vi "PicoScope3000aSettings.vi"(0 "handle in":i16, 1 "Channel A Settings":T1={"Enabled"=FALSE, "Coupling"=1, "Range"=6, "Analogue Offset"=0.0, "Bandwidth Limit"=0} {"Bandwidth Limit" items=["Full", "20MHz"]; "Range" items=["10 mV", "20 mV", "50 mV", "100 mV", "200 mV", "500 mV", "1 V", "2 V", "5 V", "10 V", "20 V", "50 V ", "100 V"]; "Coupling" items=["AC", "DC"]}, 2 "Channel B Settings":T1={"Enabled"=FALSE, "Coupling"=1, "Range"=6, "Analogue Offset"=0.0, "Bandwidth Limit"=0} {"Bandwidth Limit" items=["Full", "20MHz"]; "Range" items=["10 mV", "20 mV", "50 mV", "100 mV", "200 mV", "500 mV", "1 V", "2 V", "5 V", "10 V", "20 V", "50 V ", "100 V"]; "Coupling" items=["AC", "DC"]}, 3 "Port 0 Settings":T4={"Enabled"=FALSE, "Logic Level"=9830} {"Logic Level" items=["1.5V TTL"=9830, "2.5V CMOS"=16383]}, 5 "Trigger Settings":T3={"Trigger Enabled"=FALSE, "Trigger Source"=enum."Channel A", "Trigger Threshold (volts)"=0.0, "Trigger Direction"=2, "Trigger Delay (samples)"=0, "Auto Trigger Time (ms)"=1000} {"Trigger Direction" items=["Above", "Below", "Rising", "Falling", "Rising or Falling"]}, 7 "Max_adc":i16=32767, 9 "Device Info":T2, 11 "error in":errorcluster, 12 "Channel C Settings":T1={"Enabled"=FALSE, "Coupling"=1, "Range"=6, "Analogue Offset"=0.0, "Bandwidth Limit"=0} {"Bandwidth Limit" items=["Full", "20MHz"]; "Range" items=["10 mV", "20 mV", "50 mV", "100 mV", "200 mV", "500 mV", "1 V", "2 V", "5 V", "10 V", "20 V", "50 V ", "100 V"]; "Coupling" items=["AC", "DC"]}, 13 "Channel D Settings":T1={"Enabled"=FALSE, "Coupling"=1, "Range"=6, "Analogue Offset"=0.0, "Bandwidth Limit"=0} {"Bandwidth Limit" items=["Full", "20MHz"]; "Range" items=["10 mV", "20 mV", "50 mV", "100 mV", "200 mV", "500 mV", "1 V", "2 V", "5 V", "10 V", "20 V", "50 V ", "100 V"]; "Coupling" items=["AC", "DC"]}, 14 "Port 1 Settings":T4={"Enabled"=FALSE, "Logic Level"=9830} {"Logic Level" items=["1.5V TTL"=9830, "2.5V CMOS"=16383]}) -> (4 "handle out":i16, 8 "Enabled Array":i16[](array[numeric]), 15 "error out":errorcluster)   [LabVIEW 2010]
doc: "This VI is used to set up the oscilloscope channels and call the SetSimpleTrigger function."
uses:
  ps3000a.dll
  PicoScope3000aAnalogChannelSettings.ctl
  PicoScope3000aDigitalChannelSettings.ctl
panel:
  # "Connect to PicoScope3000aOpen.vi"
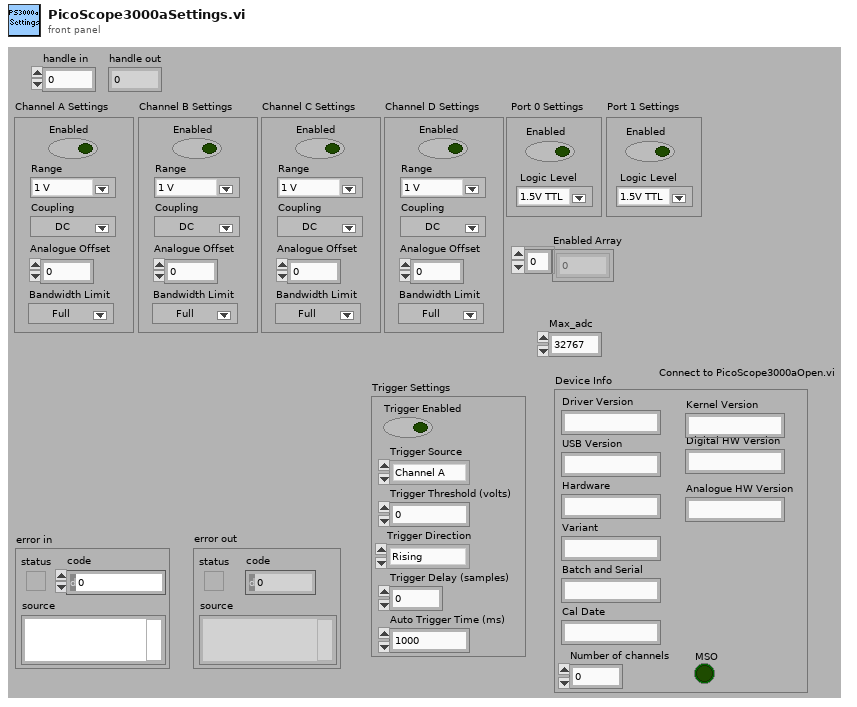
[diagram p1: front panel]
types:
  T1 = typedef "PicoScope3000aAnalogChannelSettings.ctl" = cluster{"Enabled":bool, "Coupling":u32, "Range":u32, "Analogue Offset":sgl, "Bandwidth Limit":u32}
  T2 = cluster{"Driver Version":string, "USB Version":string, "Hardware":string, "Variant":string, "Batch and Serial":string, "Cal Date":string, "Kernel Version":string, "Digital HW Version":string, "Analogue HW Version":string, "MSO":bool, "Number of channels":i16}
  T3 = cluster{"Trigger Enabled":bool, "Trigger Source":enum32{"Channel A", "Channel B", "Channel C", "Channel D", "Ext."}, "Trigger Threshold (volts)":dbl, "Trigger Direction":u32, "Trigger Delay (samples)":u32, "Auto Trigger Time (ms)":i16}
  T4 = typedef "PicoScope3000aDigitalChannelSettings.ctl" = cluster{"Enabled":bool, "Logic Level":i16}
  T5 = cluster{"status":bool, "code":u32, "source":string}
  T6 = enum32{"Channel A", "Channel B", "Channel C", "Channel D", "Ext."}
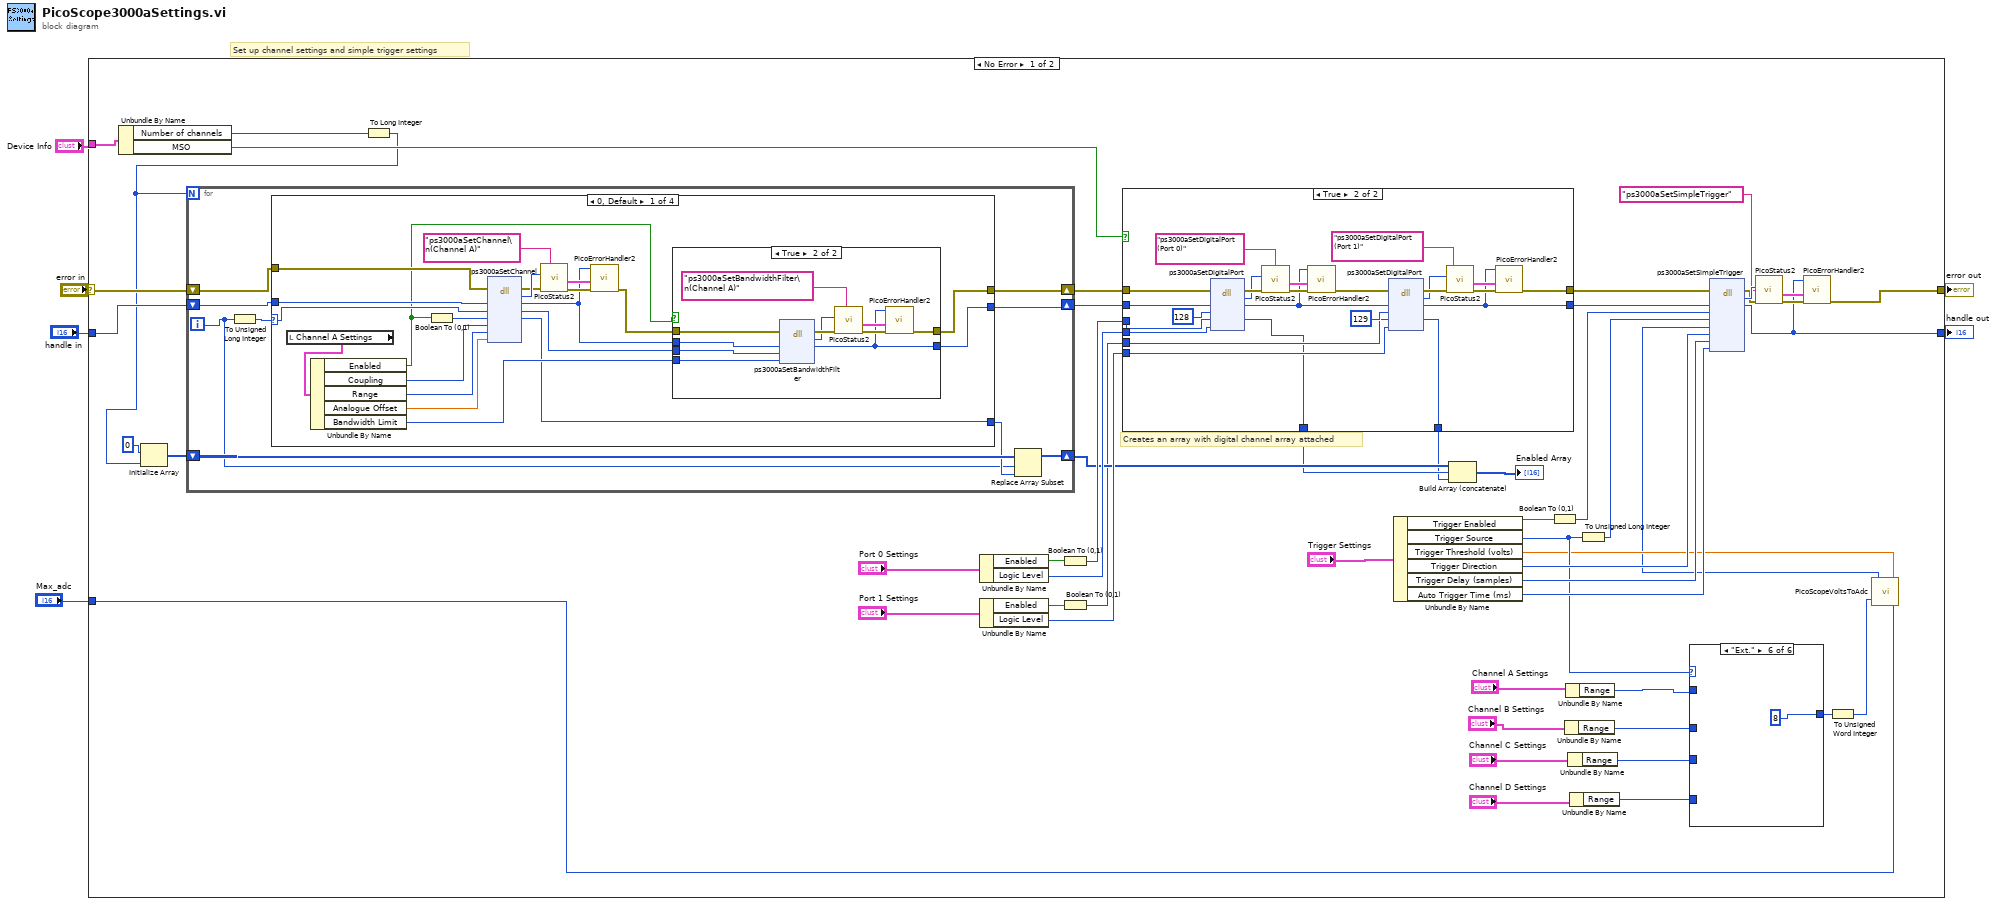
[diagram p0: block diagram]
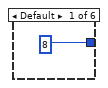
[diagram p2: hidden frame]
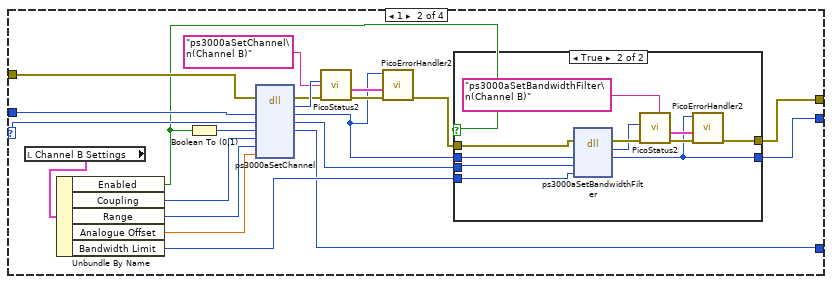
[diagram p8: hidden frame]
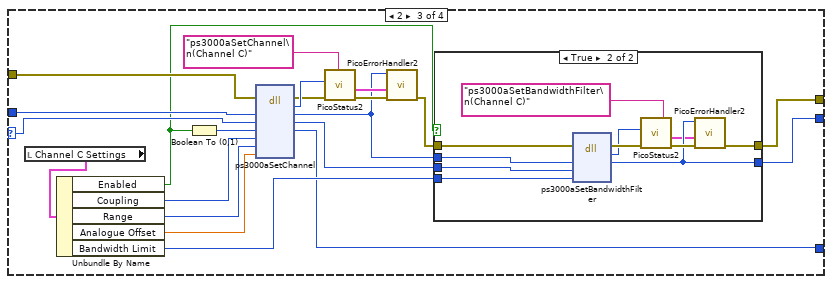
[diagram p10: hidden frame]
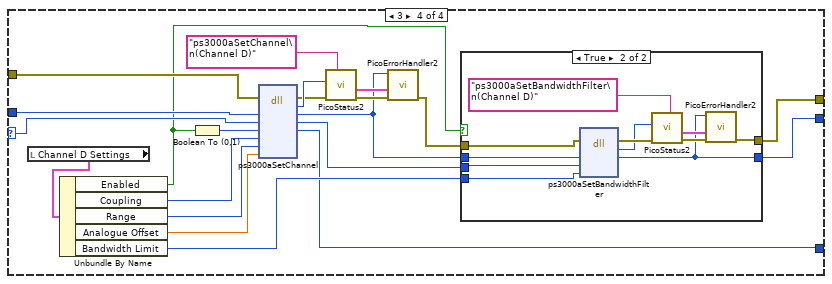
[diagram p12: hidden frame]
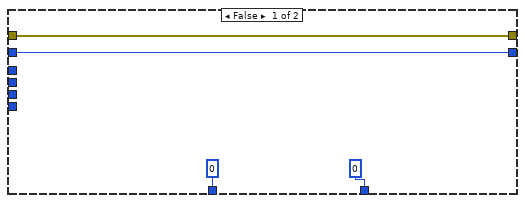
[diagram p14: hidden frame]
diagram:
  # "Set up channel settings and simple trigger settings"
  n1 = case shown="No Error" "error in" {
    selector: "error in" -> [w40 w239]
    tunnel: "handle in" -> [w39 w238]
    tunnel: [w7 w238] -> w4
    tunnel: [w50 w239] -> w3
    tunnel: "Max_adc" -> [w10 _]
    tunnel: "Device Info" -> [w28 _]
    frame No Error {
      # "Creates an array with digital channel array attached"
      n2 = Unbundle By Name(w28) -> ("Number of channels"=w27:i16, "MSO"=w26:bool)
      n3 = To Long Integer(number=w27) -> (32bit integer=w9:i32)
      n4 = Initialize Array(i16 0 ("element"), w9) -> (w32:i16[])
      n5 = for {
        N: w9 -> [_]
        shift-right: [w65] -> w38
        shift-left: w40 -> [w73]
        shift-right: [w68] -> w37
        shift-left: w39 -> [w72]
        shift-right: [w71] -> w31
        shift-left: w32 -> [w70]
        i -> [w66]
        n6 = To Unsigned Long Integer(number=w66) -> (unsigned 32bit integer=w67:u32)
        n7 = case shown="0, Default" w67 {
          selector: w67 -> [w85 w119 w153 w187]
          tunnel: w73 -> [w94 w128 w162 w196]
          tunnel: [w82 w114 w148 w182] -> w65
          tunnel: w72 -> [w93 w127 w161 w195]
          tunnel: [w81 w113 w147 w181] -> w68
          tunnel: [w80 w112 w146 w180] -> w69
          frame 0, Default {
            n8 = local read "Channel A Settings"() -> (w79:T1)
            n9 = Unbundle By Name(w79) -> ("Enabled"=w78:bool, "Coupling"=w88:u32, "Range"=w87:u32, "Analogue Offset"=w86:sgl, "Bandwidth Limit"=w83:u32)
            n10 = Boolean To (0,1)(Boolean=w78) -> (0, 1=w89:i16)
            n11 = dll-call lib="ps3000a.dll" fn="ps3000aSetChannel" ("ps3000.dll:_ps3000_open_unit@0")(error in=w94, "handle"=w93, "channel"=w85, "enabled"=w89, "dc"=w88, "range"=w87, "analogueOffset"=w86) -> (error out=w91:errorcluster, "PICO_STATUS"=w92:u32, "handle"=w75:i16, "channel"=w84:u32, "enabled"=w80:i16)  [unwired: 5 in, 1 out]
            n12 = call "PicoStatus2.vi"("PICO source"="ps3000aSetChannel\n(Channel A)" ("source"), "Error in"=w91, "PICO STATUS"=w92) -> ("error out"=w77:errorcluster, "PICO_STATUS out"=w76:T5)  [unwired: 5 in]
            n13 = call "PicoErrorHandler2.vi"("error in (no error)"=w77, "PICO_STATUS in"=w76, "handle In"=w75) -> ("error out"=w74:errorcluster)  [unwired: 8 in]
            n14 = case shown="True" w78 {
              tunnel: w75 -> [w95 w106]
              tunnel: w74 -> [w96 w105]
              tunnel: w84 -> [_ w104]
              tunnel: w83 -> [_ w103]
              tunnel: [w96 w99] -> w82
              tunnel: [w95 w97] -> w81
              frame False {
              }
              frame True {
                n15 = dll-call lib="ps3000a.dll" fn="ps3000aSetBandwidthFilter" ("ps3000.dll:_ps3000_open_unit@0")(error in=w105, "handle"=w106, "channel"=w104, "bandwidth"=w103) -> (error out=w107:errorcluster, "PICO_STATUS"=w102:u32, "handle"=w97:i16)  [unwired: 4 in, 1 out]
                n16 = call "PicoStatus2.vi"("PICO source"="ps3000aSetBandwidthFilter\n(Channel A)" ("source"), "Error in"=w107, "PICO STATUS"=w102) -> ("error out"=w100:errorcluster, "PICO_STATUS out"=w98:T5)  [unwired: 5 in]
                n17 = call "PicoErrorHandler2.vi"("error in (no error)"=w100, "PICO_STATUS in"=w98, "handle In"=w97) -> ("error out"=w99:errorcluster)  [unwired: 8 in]
              }
            }
          }
          frame 1 {
            n18 = local read "Channel B Settings"() -> (w118:T1)
            n19 = Unbundle By Name(w118) -> ("Enabled"=w115:bool, "Coupling"=w122:u32, "Range"=w121:u32, "Analogue Offset"=w120:sgl, "Bandwidth Limit"=w116:u32)
            n20 = Boolean To (0,1)(Boolean=w115) -> (0, 1=w123:i16)
            n21 = dll-call lib="ps3000a.dll" fn="ps3000aSetChannel" ("ps3000.dll:_ps3000_open_unit@0")(error in=w128, "handle"=w127, "channel"=w119, "enabled"=w123, "dc"=w122, "range"=w121, "analogueOffset"=w120) -> (error out=w125:errorcluster, "PICO_STATUS"=w126:u32, "handle"=w109:i16, "channel"=w117:u32, "enabled"=w112:i16)  [unwired: 5 in, 1 out]
            n22 = call "PicoStatus2.vi"("PICO source"="ps3000aSetChannel\n(Channel B)" ("source"), "Error in"=w125, "PICO STATUS"=w126) -> ("error out"=w111:errorcluster, "PICO_STATUS out"=w110:T5)  [unwired: 5 in]
            n23 = call "PicoErrorHandler2.vi"("error in (no error)"=w111, "PICO_STATUS in"=w110, "handle In"=w109) -> ("error out"=w108:errorcluster)  [unwired: 8 in]
            n24 = case shown="True" w115 {
              tunnel: w109 -> [w129 w140]
              tunnel: w108 -> [w130 w139]
              tunnel: w117 -> [_ w138]
              tunnel: w116 -> [_ w137]
              tunnel: [w130 w133] -> w114
              tunnel: [w129 w131] -> w113
              frame False {
              }
              frame True {
                n25 = dll-call lib="ps3000a.dll" fn="ps3000aSetBandwidthFilter" ("ps3000.dll:_ps3000_open_unit@0")(error in=w139, "handle"=w140, "channel"=w138, "bandwidth"=w137) -> (error out=w141:errorcluster, "PICO_STATUS"=w136:u32, "handle"=w131:i16)  [unwired: 4 in, 1 out]
                n26 = call "PicoStatus2.vi"("PICO source"="ps3000aSetBandwidthFilter\n(Channel B)" ("source"), "Error in"=w141, "PICO STATUS"=w136) -> ("error out"=w134:errorcluster, "PICO_STATUS out"=w132:T5)  [unwired: 5 in]
                n27 = call "PicoErrorHandler2.vi"("error in (no error)"=w134, "PICO_STATUS in"=w132, "handle In"=w131) -> ("error out"=w133:errorcluster)  [unwired: 8 in]
              }
            }
          }
          frame 2 {
            n28 = local read "Channel C Settings"() -> (w152:T1)
            n29 = Unbundle By Name(w152) -> ("Enabled"=w149:bool, "Coupling"=w156:u32, "Range"=w155:u32, "Analogue Offset"=w154:sgl, "Bandwidth Limit"=w150:u32)
            n30 = Boolean To (0,1)(Boolean=w149) -> (0, 1=w157:i16)
            n31 = dll-call lib="ps3000a.dll" fn="ps3000aSetChannel" ("ps3000.dll:_ps3000_open_unit@0")(error in=w162, "handle"=w161, "channel"=w153, "enabled"=w157, "dc"=w156, "range"=w155, "analogueOffset"=w154) -> (error out=w159:errorcluster, "PICO_STATUS"=w160:u32, "handle"=w143:i16, "channel"=w151:u32, "enabled"=w146:i16)  [unwired: 5 in, 1 out]
            n32 = call "PicoStatus2.vi"("PICO source"="ps3000aSetChannel\n(Channel C)" ("source"), "Error in"=w159, "PICO STATUS"=w160) -> ("error out"=w145:errorcluster, "PICO_STATUS out"=w144:T5)  [unwired: 5 in]
            n33 = call "PicoErrorHandler2.vi"("error in (no error)"=w145, "PICO_STATUS in"=w144, "handle In"=w143) -> ("error out"=w142:errorcluster)  [unwired: 8 in]
            n34 = case shown="True" w149 {
              tunnel: w143 -> [w163 w174]
              tunnel: w142 -> [w164 w173]
              tunnel: w151 -> [_ w172]
              tunnel: w150 -> [_ w171]
              tunnel: [w164 w167] -> w148
              tunnel: [w163 w166] -> w147
              frame False {
              }
              frame True {
                n35 = dll-call lib="ps3000a.dll" fn="ps3000aSetBandwidthFilter" ("ps3000.dll:_ps3000_open_unit@0")(error in=w173, "handle"=w174, "channel"=w172, "bandwidth"=w171) -> (error out=w175:errorcluster, "PICO_STATUS"=w170:u32, "handle"=w166:i16)  [unwired: 4 in, 1 out]
                n36 = call "PicoStatus2.vi"("PICO source"="ps3000aSetBandwidthFilter\n(Channel C)" ("source"), "Error in"=w175, "PICO STATUS"=w170) -> ("error out"=w168:errorcluster, "PICO_STATUS out"=w165:T5)  [unwired: 5 in]
                n37 = call "PicoErrorHandler2.vi"("error in (no error)"=w168, "PICO_STATUS in"=w165, "handle In"=w166) -> ("error out"=w167:errorcluster)  [unwired: 8 in]
              }
            }
          }
          frame 3 {
            n38 = local read "Channel D Settings"() -> (w186:T1)
            n39 = Unbundle By Name(w186) -> ("Enabled"=w183:bool, "Coupling"=w190:u32, "Range"=w189:u32, "Analogue Offset"=w188:sgl, "Bandwidth Limit"=w184:u32)
            n40 = Boolean To (0,1)(Boolean=w183) -> (0, 1=w191:i16)
            n41 = dll-call lib="ps3000a.dll" fn="ps3000aSetChannel" ("ps3000.dll:_ps3000_open_unit@0")(error in=w196, "handle"=w195, "channel"=w187, "enabled"=w191, "dc"=w190, "range"=w189, "analogueOffset"=w188) -> (error out=w193:errorcluster, "PICO_STATUS"=w194:u32, "handle"=w177:i16, "channel"=w185:u32, "enabled"=w180:i16)  [unwired: 5 in, 1 out]
            n42 = call "PicoStatus2.vi"("PICO source"="ps3000aSetChannel\n(Channel D)" ("source"), "Error in"=w193, "PICO STATUS"=w194) -> ("error out"=w179:errorcluster, "PICO_STATUS out"=w178:T5)  [unwired: 5 in]
            n43 = call "PicoErrorHandler2.vi"("error in (no error)"=w179, "PICO_STATUS in"=w178, "handle In"=w177) -> ("error out"=w176:errorcluster)  [unwired: 8 in]
            n44 = case shown="True" w183 {
              tunnel: w177 -> [w197 w208]
              tunnel: w176 -> [w198 w207]
              tunnel: w185 -> [_ w206]
              tunnel: w184 -> [_ w205]
              tunnel: [w198 w199] -> w182
              tunnel: [w197 w200] -> w181
              frame False {
              }
              frame True {
                n45 = dll-call lib="ps3000a.dll" fn="ps3000aSetBandwidthFilter" ("ps3000.dll:_ps3000_open_unit@0")(error in=w207, "handle"=w208, "channel"=w206, "bandwidth"=w205) -> (error out=w209:errorcluster, "PICO_STATUS"=w204:u32, "handle"=w200:i16)  [unwired: 4 in, 1 out]
                n46 = call "PicoStatus2.vi"("PICO source"="ps3000aSetBandwidthFilter\n(Channel D)" ("source"), "Error in"=w209, "PICO STATUS"=w204) -> ("error out"=w202:errorcluster, "PICO_STATUS out"=w201:T5)  [unwired: 5 in]
                n47 = call "PicoErrorHandler2.vi"("error in (no error)"=w202, "PICO_STATUS in"=w201, "handle In"=w200) -> ("error out"=w199:errorcluster)  [unwired: 8 in]
              }
            }
          }
        }
        n48 = Replace Array Subset(array=w70, new element=w69, index=w66) -> (w71:i16[])
      }
      n49 = Unbundle By Name("Port 0 Settings") -> ("Enabled"=w48:bool, "Logic Level"=w47:i16)
      n50 = Unbundle By Name("Port 1 Settings") -> ("Enabled"=w45:bool, "Logic Level"=w44:i16)
      n51 = Boolean To (0,1)(Boolean=w48) -> (0, 1=w35:i16)
      n52 = Boolean To (0,1)(Boolean=w45) -> (0, 1=w30:i16)
      n53 = case shown="True" w26 {
        tunnel: w37 -> [w212 w237]
        tunnel: w35 -> [_ w235]
        tunnel: w47 -> [_ w234]
        tunnel: w30 -> [_ w228]
        tunnel: w44 -> [_ w227]
        tunnel: [w212 w216] -> w43
        tunnel: [w213 w217] -> w42
        tunnel: w38 -> [w213 w226]
        tunnel: [i16 0 ("enabled") w223] -> w15
        tunnel: [i16 0 ("enabled") w222] -> w14
        frame False {
        }
        frame True {
          n54 = dll-call lib="PS3000a.dll" fn="ps3000aSetDigitalPort"(error in=w226, "handle"=w237, "port"=u32 128, "enabled"=w235, "logicLevel"=w234) -> (error out=w233:errorcluster, "PICO_STATUS"=w225:u32, "handle"=w215:i16, "enabled"=w223:i16)  [unwired: 4 in, 1 out]
          n55 = call "PicoStatus2.vi"("PICO source"="ps3000aSetDigitalPort (Port 0)" ("source"), "Error in"=w233, "PICO STATUS"=w225) -> ("error out"=w221:errorcluster, "PICO_STATUS out"=w218:T5)  [unwired: 5 in]
          n56 = call "PicoErrorHandler2.vi"("error in (no error)"=w221, "PICO_STATUS in"=w218, "handle In"=w215) -> ("error out"=w214:errorcluster)  [unwired: 8 in]
          n57 = dll-call lib="PS3000a.dll" fn="ps3000aSetDigitalPort"(error in=w214, "handle"=w215, "port"=u32 129, "enabled"=w228, "logicLevel"=w227) -> (error out=w232:errorcluster, "PICO_STATUS"=w224:u32, "handle"=w216:i16, "enabled"=w222:i16)  [unwired: 4 in, 1 out]
          n58 = call "PicoStatus2.vi"("PICO source"="ps3000aSetDigitalPort (Port 1)" ("source"), "Error in"=w232, "PICO STATUS"=w224) -> ("error out"=w220:errorcluster, "PICO_STATUS out"=w219:T5)  [unwired: 5 in]
          n59 = call "PicoErrorHandler2.vi"("error in (no error)"=w220, "PICO_STATUS in"=w219, "handle In"=w216) -> ("error out"=w217:errorcluster)  [unwired: 8 in]
        }
      }
      n60 = Unbundle By Name("Trigger Settings") -> ("Trigger Enabled"=w56:bool, "Trigger Source"=w25:T6, "Trigger Threshold (volts)"=w24:dbl, "Trigger Direction"=w41:u32, "Trigger Delay (samples)"=w58:u32, "Auto Trigger Time (ms)"=w57:i16)
      n61 = Build Array (concatenate)(w31, w15, w14) -> (→"Enabled Array":i16[])
      n62 = Boolean To (0,1)(Boolean=w56) -> (0, 1=w55:i16)
      n63 = Unbundle By Name("Channel B Settings") -> ("Range"=w21:u32)
      n64 = Unbundle By Name("Channel A Settings") -> ("Range"=w18:u32)
      n65 = Unbundle By Name("Channel C Settings") -> ("Range"=w20:u32)
      n66 = Unbundle By Name("Channel D Settings") -> ("Range"=w19:u32)
      n67 = To Unsigned Long Integer(number=w25) -> (unsigned 32bit integer=w36:u32)
      n68 = case shown="\"Ext.\"" w25 {
        tunnel: w18 -> [_ w60 _ _ _ _]
        tunnel: w21 -> [_ _ w61 _ _ _]
        tunnel: w20 -> [_ _ _ w62 _ _]
        tunnel: w19 -> [_ _ _ _ w63 _]
        tunnel: [u32 8 ("Range") w60 w61 w62 w63 u32 8] -> w16
        frame Default {
        }
        frame "Channel A" {
        }
        frame "Channel B" {
        }
        frame "Channel C" {
        }
        frame "Channel D" {
        }
        frame "Ext." {
        }
      }
      n69 = To Unsigned Word Integer(number=w16) -> (unsigned 16bit integer=w17:u16)
      n70 = call "PicoScopeVoltsToAdc.vi"("Max_adc"=w10, "Units"=w24, "Range Index"=w17) -> ("ADC count"=w23:i16)
      n71 = dll-call lib="ps3000a.dll" fn="ps3000aSetSimpleTrigger" ("ps3000.dll:_ps3000_open_unit@0")(error in=w42, "handle"=w43, "enabled"=w55, "source"=w36, "threshold"=w23, "direction"=w41, "delay"=w58, "autoTrigger_ms"=w57) -> (error out=w53:errorcluster, "PICO_STATUS"=w54:u32, "handle"=w7:i16)  [unwired: 8 in, 1 out]
      n72 = call "PicoStatus2.vi"("PICO source"="ps3000aSetSimpleTrigger" ("source"), "Error in"=w53, "PICO STATUS"=w54) -> ("error out"=w51:errorcluster, "PICO_STATUS out"=w8:T5)  [unwired: 5 in]
      n73 = call "PicoErrorHandler2.vi"("error in (no error)"=w51, "PICO_STATUS in"=w8, "handle In"=w7) -> ("error out"=w50:errorcluster)  [unwired: 8 in]
    }
    frame Error {
    }
  }
  "handle out" <- w4
  "error out" <- w3
